vi "BuildCall.vi"(7 "PythonConverter_BD in":refnum<class "PyConvBD.lvclass">, 8 "error in":errorcluster, 11 "FlatSequenceFrame in":refnum<class "FlatSequenceFrame.lvclass">) -> (0 "error out":errorcluster, 3 "FlatSequenceFrame out":refnum<class "FlatSequenceFrame.lvclass">, 5 "PythonConverter_BD out":refnum<class "PyConvBD.lvclass">)   [LabVIEW 2014, in "FlatSequenceFrame.lvclass"]
uses:
  FlatSequenceFrame.lvclass
  Python/PythonConverter_BD/PyConvBD.lvclass
  Python/PythonConverter_BD/TypeDefs/NodeCall_TD.ctl
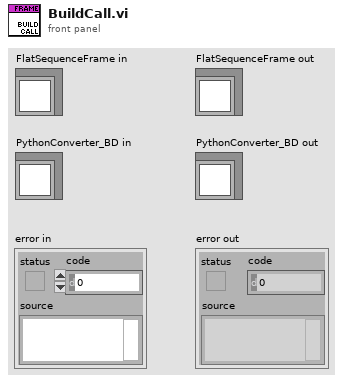
[diagram p1: front panel]
types:
  T1 = typedef "NodeCall_TD.ctl" = cluster{"call":string, "collect":string, "Threaded":bool, "branches":string[]}
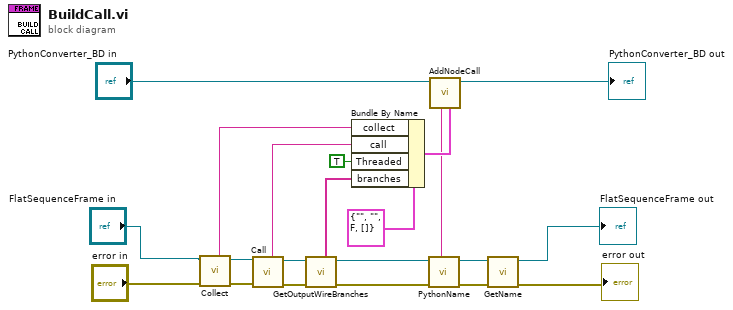
[diagram p0: block diagram]
diagram:
  n1 = call-dynamic "Collect.vi"("error in"="error in", "FlatSequenceFrame in"="FlatSequenceFrame in") -> ("error out"=w7:errorcluster, "FlatSequenceFrame out"=w8:refnum<class "FlatSequenceFrame.lvclass">, "collect"=w12:string)  [unwired: 5 in]
  n2 = call-dynamic "Call.vi"("error in"=w7, "FlatSequenceFrame in"=w8) -> ("error out"=w3:errorcluster, "FlatSequenceFrame out"=w5:refnum<class "FlatSequenceFrame.lvclass">, "call"=w6:string)  [unwired: 5 in]
  n3 = call-dynamic "GetOutputWireBranches.vi"("error in"=w3, "FlatSequenceFrame in"=w5) -> ("error out"=w1:errorcluster, "FlatSequenceFrame out"=w2:refnum<class "FlatSequenceFrame.lvclass">, "branches"=w4:string[])  [unwired: 5 in]
  n4 = Bundle By Name(cluster=T1 {"call"="", "collect"="", "Threaded"=FALSE, "branches"=[]} ("call"), "collect"=w12, "call"=w6, "Threaded"=TRUE, "branches"=w4) -> (w21:T1)
  n5 = call-dynamic "PythonName.vi"("error in"=w1, "FlatSequenceFrame in"=w2) -> ("error out"=w9:errorcluster, "FlatSequenceFrame out"=w10:refnum<class "FlatSequenceFrame.lvclass">, "UID"=w11:string)  [unwired: 6 in, 1 out]
  n6 = call "AddNodeCall.vi"("call"=w21, "name"=w11, "PythonConverter_BD in"="PythonConverter_BD in") -> ("PythonConverter_BD out"=→"PythonConverter_BD out":refnum<class "PyConvBD.lvclass">)  [unwired: 5 in, 1 out]
  n7 = call-dynamic "GetName.vi"("error in"=w9, "FlatSequenceFrame in"=w10) -> ("error out"=→"error out":errorcluster, "FlatSequenceFrame out"=→"FlatSequenceFrame out":refnum<class "FlatSequenceFrame.lvclass">)  [unwired: 4 in, 2 out]
